vi "maxigauge_test.vi"(5 "maxi_delay 3":u32=100, 6 "err_in":errorcluster, 7 "maxi_delay":u32=100, 9 "?":i32=1, 10 "maxi_visa":refnum<visa-resource-name>="COM8") -> (0 "err_out":errorcluster, 2 "pressure":dbl, 3 "Pressure (Torr)":string)   [LabVIEW 2019]
uses:
  <vilib>/Instr/_visa.llb/VISA Configure Serial Port (Instr).vi
panel:
  out "return count 2":u32
  out "return count":u32
  out "read_2":string
  out "read_1":string
  out "Overall Status":bool
  out "Acknowledgement Status":bool
  # "Sensor Number"
  # "VISA"
  # "DELAY"
  # "BYTE AT PORT"
  # "STATUS"
  # "ERROR"
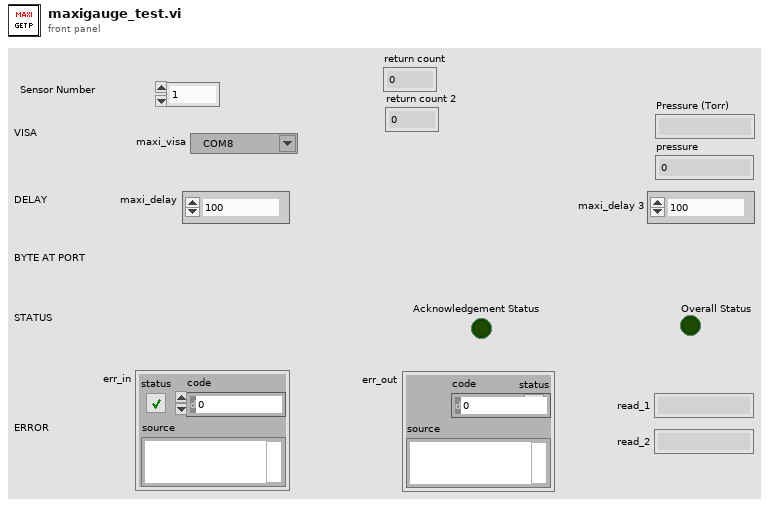
[diagram p1: front panel]
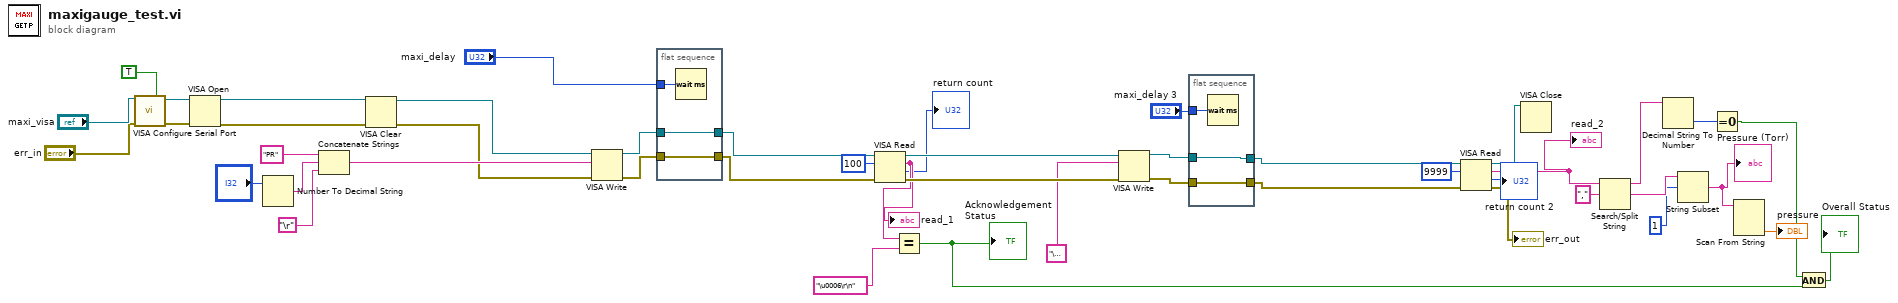
[diagram p0: block diagram]
diagram:
  n1 = call-poly "VISA Configure Serial Port"("VISA resource name"="maxi_visa", "Enable Termination\nChar (T)"=TRUE ("Enable Termination\nChar (T)"), "error in (no error)"="err_in") -> ("VISA resource name out"=w10:refnum<visa-resource-name>, "error out"=w9:errorcluster)  [unwired: 11 in]
  n2 = VISA Open(error in (no error)=w9, VISA resource name=w10) -> (VISA resource name=w12:refnum<visa-resource-name>, error out=w11:errorcluster)  [unwired: 3 in]
  n3 = Number To Decimal String(number="?") -> (decimal integer string=w19:string)  [unwired: 1 in]
  n4 = Concatenate Strings("PR" ("string"), w19, "\r") -> (w20:string)
  n5 = VISA Clear(VISA resource name=w12, error in (no error)=w11) -> (VISA resource name out=w15:refnum<visa-resource-name>, error out=w14:errorcluster)
  n6 = VISA Write(VISA resource name=w15, write buffer=w20, error in (no error)=w14) -> (VISA resource name out=w44:refnum<visa-resource-name>, error out=w46:errorcluster)  [unwired: 1 out]
  n7 = flat-sequence {
    tunnel: w46 -> [w48]
    tunnel: [w48] -> w45
    tunnel: w44 -> [w47]
    tunnel: [w47] -> w43
    tunnel: "maxi_delay" -> [w49]
    frame #0 {
      n8 = Wait (ms)(milliseconds to wait=w49) -> ()  [unwired: 1 out]
    }
  }
  n9 = VISA Read(VISA resource name=w43, byte count=u32 100, error in (no error)=w45) -> (VISA resource name out=w41:refnum<visa-resource-name>, read buffer=w26:string, return count=→"return count":u32, error out=w40:errorcluster)
  "read_1" <- w26
  n10 = Equal?(x=w26, y="\u0006\r\n") -> (x = y?=w23:bool)
  "Acknowledgement Status" <- w23
  n11 = VISA Write(VISA resource name=w41, write buffer="\u0005", error in (no error)=w40) -> (VISA resource name out=w37:refnum<visa-resource-name>, error out=w36:errorcluster)  [unwired: 1 out]
  n12 = flat-sequence {
    tunnel: [w51] -> w39
    tunnel: [w52] -> w38
    tunnel: w37 -> [w52]
    tunnel: w36 -> [w51]
    tunnel: "maxi_delay 3" -> [w50]
    frame #0 {
      n13 = Wait (ms)(milliseconds to wait=w50) -> ()  [unwired: 1 out]
    }
  }
  n14 = VISA Read(VISA resource name=w38, byte count=u32 9999, error in (no error)=w39) -> (VISA resource name out=w6:refnum<visa-resource-name>, read buffer=w33:string, return count=→"return count 2":u32, error out=→"err_out":errorcluster)
  "read_2" <- w33
  n15 = VISA Close(VISA resource name=w6) -> ()  [unwired: 1 in, 1 out]
  n16 = Search/Split String(string=w33, search string/char (-)=",") -> (substring before match=w29:string, match + rest of string=w31:string)  [unwired: 1 in, 1 out]
  n17 = Decimal String To Number(string=w29) -> (number=w28:i32)  [unwired: 2 in, 1 out]
  n18 = String Subset(string=w31, offset (0)=1) -> (substring=w17:string)  [unwired: 1 in]
  "Pressure (Torr)" <- w17
  n19 = Equal To 0?(x=w28) -> (x = 0?=w24:bool)
  n20 = Scan From String(input string=w17) -> (output 1=→"pressure":dbl)  [unwired: 4 in, 3 out]
  n21 = And(x=w24, y=w23) -> (x .and. y?=→"Overall Status":bool)
